vi "Initialize Grips Robot.vi"(4 "Name":string, 6 "JointMapping":T1, 8 "error in (no error)":errorcluster, 9 "hw interface":T4, 10 "kinematic_parameters":T3, 11 "Grips Robot in":refnum<class "Grips Robot.lvclass">) -> (0 "error out":errorcluster, 3 "Grips Robot out":refnum<class "Grips Robot.lvclass">)   [LabVIEW 2013, in "Grips Robot.lvclass"]
uses:
  Grips Robot.lvclass
  <vilib>/robotics/Kinematics/Link/Joint Type.ctl
  JointMapping.ctl
  Grips Robot.lvclass/Grips Robot.ctl
  Hardware Interface/Hardware Interface.lvclass/Hardware Interface.ctl
  robotic_arm_labview/Kinematics/Robot/Robot Arm.lvclass
  Hardware Interface/Hardware Interface.lvclass
  <vilib>/robotics/Kinematics/Link/NI_Robotics_Link.lvclass
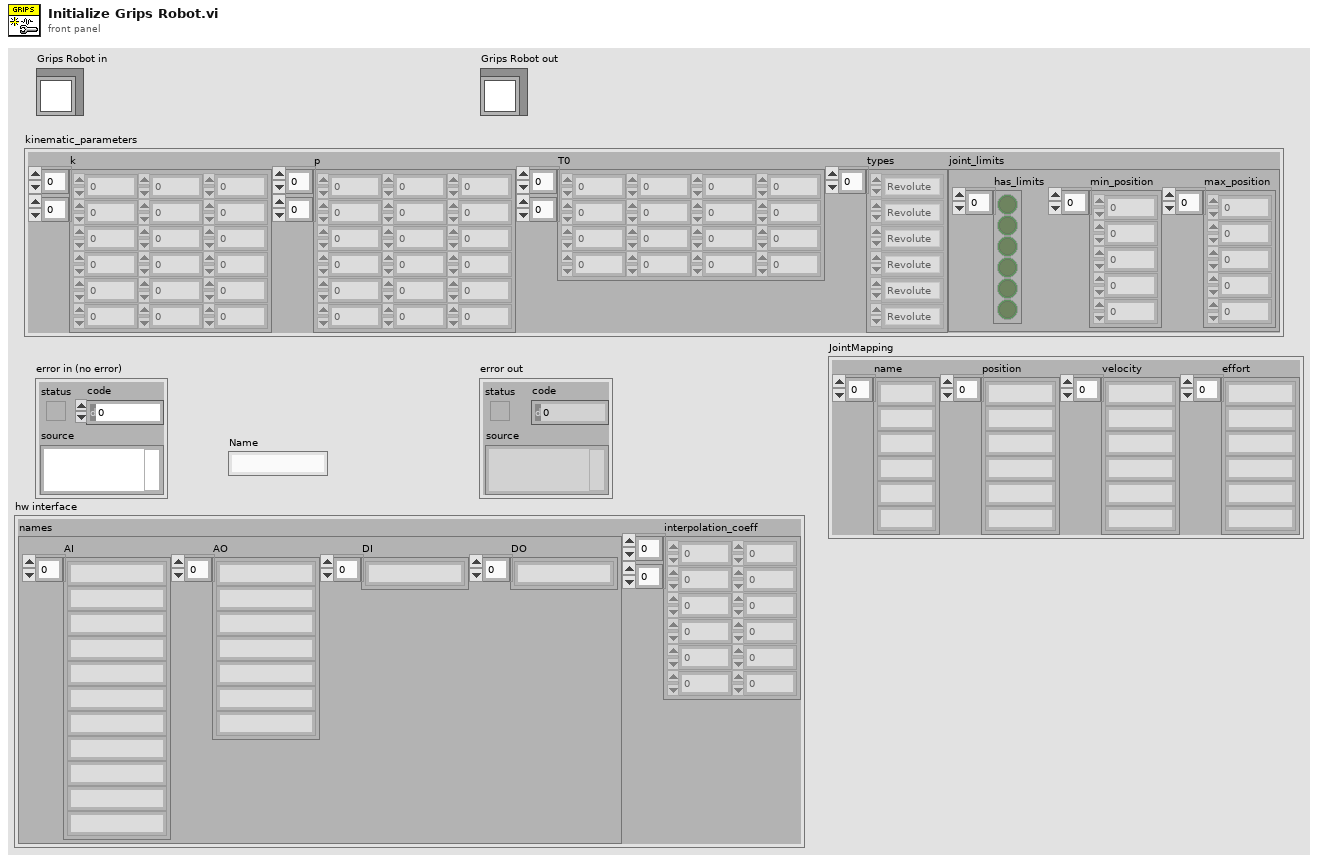
[diagram p1: front panel]
types:
  T1 = typedef "JointMapping.ctl" = cluster{"name":string[], "position":string[], "velocity":string[], "effort":string[]}
  T2 = typedef "NI_Robotics_Link.lvclass/Joint Type.ctl" = enum16{"Revolute", "Prismatic"}
  T3 = cluster{"k":sgl[][], "p":sgl[][], "T0":sgl[][], "types":T2[], "joint_limits":cluster{"has_limits":bool[], "min_position":sgl[], "max_position":sgl[]}}
  T4 = cluster{"names":cluster{"AI":string[], "AO":string[], "DI":string[], "DO":string[]}, "interpolation_coeff":sgl[][]}
  T5 = cluster{"has_limits":bool[], "min_position":sgl[], "max_position":sgl[]}
  T6 = cluster{"k":dbl[], "p":dbl[], "joint type":T2, "joint coordinate offset":dbl}
  T7 = cluster{"AI":string[], "AO":string[], "DI":string[], "DO":string[]}
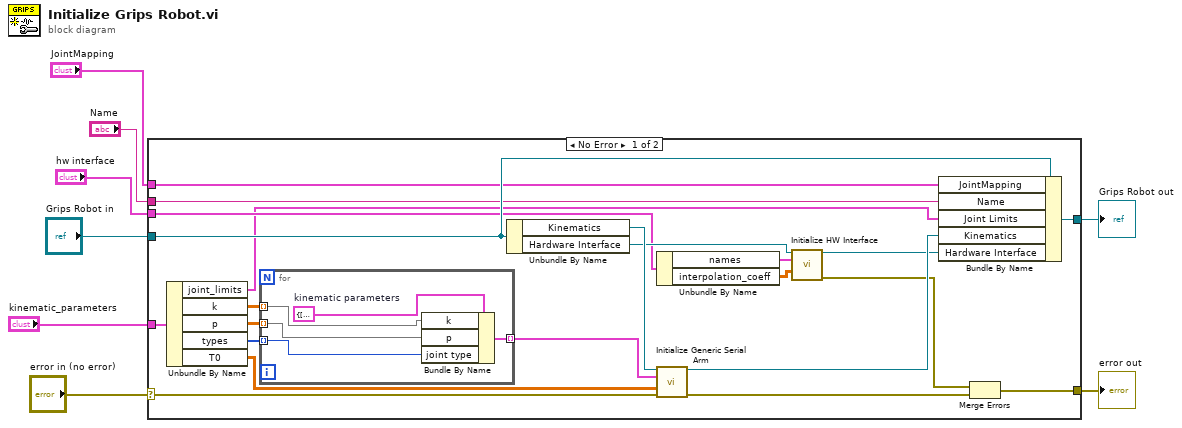
[diagram p0: block diagram]
diagram:
  n1 = case shown="No Error" "error in (no error)" {
    selector: "error in (no error)" -> [w30 w37]
    tunnel: [w21 w37] -> w7
    tunnel: [w27 w36] -> w5
    tunnel: "Grips Robot in" -> [w28 w36]
    tunnel: "hw interface" -> [w20 _]
    tunnel: "kinematic_parameters" -> [w17 _]
    tunnel: "Name" -> [w10 _]
    tunnel: "JointMapping" -> [w9 _]
    frame No Error {
      n2 = Unbundle By Name(w17) -> ("joint_limits"=w11:T5, "k"=w14:sgl[][], "p"=w15:sgl[][], "types"=w16:T2[], "T0"=w12:sgl[][])
      n3 = for {
        tunnel: w16 -> [w34] mode=indexing
        tunnel: w15 -> [w33] mode=indexing
        tunnel: w14 -> [w32] mode=indexing
        tunnel: [w31] -> w13 mode=indexing
        w35 = T6 {"k"=[], "p"=[], "joint type"=enum."Prismatic", "joint coordinate offset"=0.0}  # kinematic parameters
        n4 = Bundle By Name(cluster=w35, "k"=w32, "p"=w33, "joint type"=w34) -> (w31:T6)
      }
      n5 = Unbundle By Name(w28) -> ("Kinematics"=w29:refnum<class "Robot Arm.lvclass">, "Hardware Interface"=w25:refnum<class "Hardware Interface.lvclass">)
      n6 = Unbundle By Name(w20) -> ("names"=w19:T7, "interpolation_coeff"=w18:sgl[][])
      n7 = call "Initialize Generic Serial Arm.vi"("Robot Arm in"=w29, "kinematic parameters"=w13, "Home Transform T0"=w12, "error in (no error)"=w30) -> ("Robot Arm out"=w26:refnum<class "Robot Arm.lvclass">, "error out"=w22:errorcluster)  [unwired: 10 in]
      n8 = call "Initialize HW Interface.vi"("Hardware Interface in"=w25, "HW Interface Names"=w19, "Interpolation Coefficients"=w18) -> ("Hardware Interface out"=w24:refnum<class "Hardware Interface.lvclass">, "error out"=w23:errorcluster)  [unwired: 11 in]
      n9 = Bundle By Name(cluster=w28, "JointMapping"=w9, "Name"=w10, "Joint Limits"=w11, "Kinematics"=w26, "Hardware Interface"=w24) -> (w27:refnum<class "Grips Robot.lvclass">)
      n10 = Merge Errors(w23, w22) -> (w21:errorcluster)
    }
    frame Error {
    }
  }
  "error out" <- w7
  "Grips Robot out" <- w5
